vi "catch.vi"(11 "NXT/EV3":T1) -> (3 "NXT/EV3 2":T1)   [LabVIEW 2016]
uses:
  <vilib>/NXT/Subs/LVHSConnector.ctl
  <vilib>/NXT/LegoClasses/BrickReference/BrickReference.lvclass
  <vilib>/NXT/NXT Controls/ConnectionType.ctl
  <vilib>/NXT/Block Support/NXT_OutputPort.ctl
  <vilib>/NXT/NXTIO Xnodes/NXTIONodeSubVIs/NXTMoveMotors.vi
  <vilib>/NXT/Dual Mode Library/Waits/Wait_Num.vi
  <vilib>/NXT/NXTIO Xnodes/NXTIONodeSubVIs/NXTStopMotors.vi
  <vilib>/NXT/Dual Mode Library/Waits/Wait_Rotation.vi
  <vilib>/NXT/NXTIO Xnodes/AddressXNode/NXTIOAddress.xnode
  <vilib>/NXT/NXTIO Xnodes/NXTIOXNode/NXTIO.xnode
panel:
  in  "Numeric":dbl format="%#1.6f"
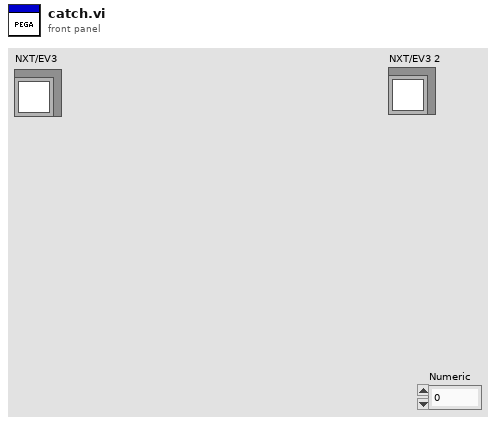
[diagram p1: front panel]
types:
  T1 = typedef "LVHSConnector.ctl" = refnum<class "BrickReference.lvclass">
  T2 = typedef "ConnectionType.ctl" = enum16{"Bluetooth", "USB", "WiFi"}
  T3 = typedef "NXT_OutputPort.ctl" = u8
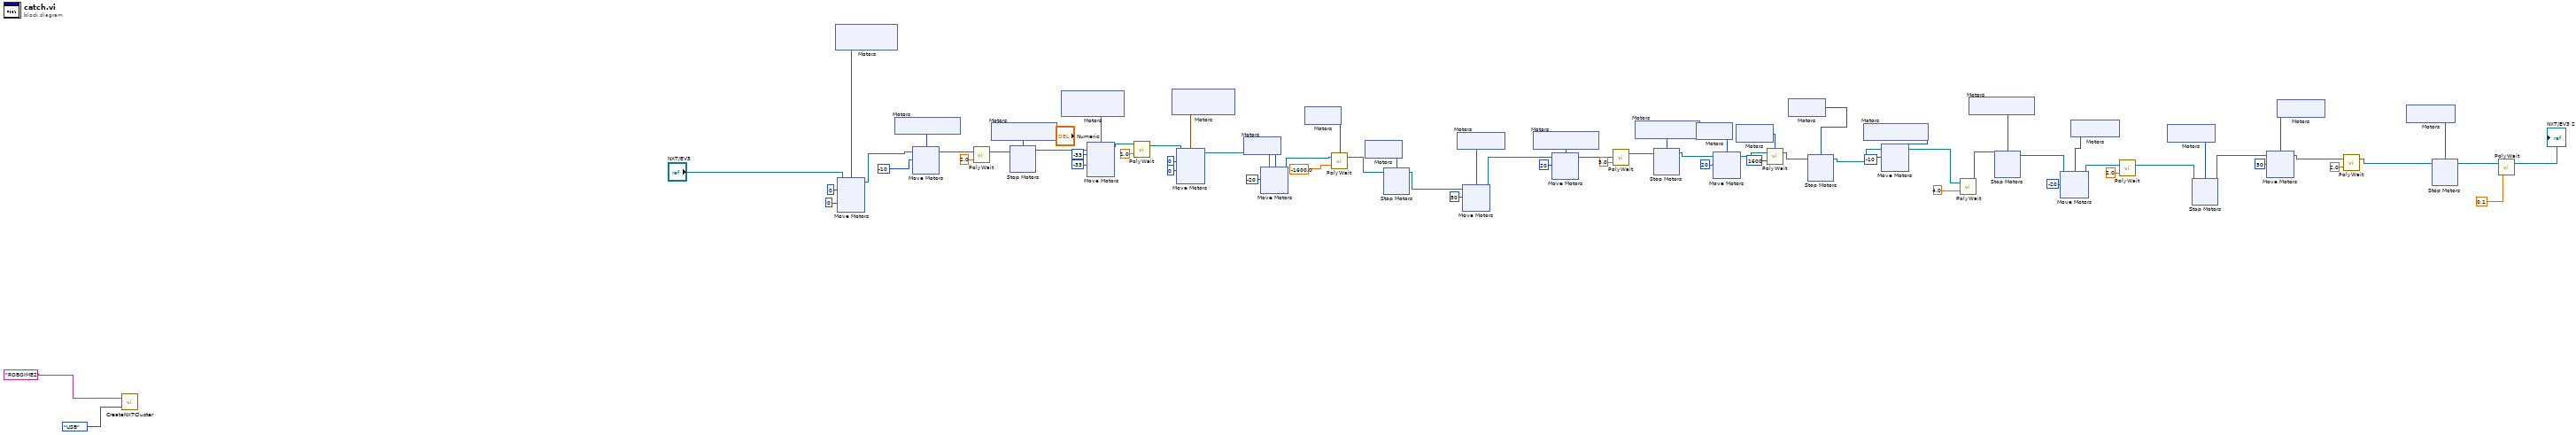
[diagram p0: block diagram]
diagram:
  n1 = call <vilib>:"CreateNXTCluster.vi"("Connection Type"=ConnectionType."USB", "NXT/EV3 name"="ROBOIME2") -> ()  [unwired: 2 in, 1 out]
  n2 = xnode "Motors"() -> ("Motor"=w20:cluster{"Port":T3, "Port":T3})
  n3 = xnode "Move Motors"("Power/Speed 2"=i8 0 ("Power/Speed 1"), "Power/Speed 1"=i8 0, "Motors"=w20, "NXT/EV3"="NXT/EV3") -> ("NXT/EV3"=w71:T1)
  n4 = xnode "Motors"() -> ("Motor"=w69:T3)
  n5 = xnode "Move Motors"("Power/Speed 1"=i8 -10, "Motors"=w69, "NXT/EV3"=w71) -> ("NXT/EV3"=w66:T1)
  n6 = call-poly <vilib>:"PolyWait.vi"("Time (1 sec)"=sgl 2.0, "NXT/EV3"=w66) -> ("NXT/EV3"=w65:T1)  [unwired: 2 in]
  n7 = xnode "Motors"() -> ("Motor"=w58:T3)
  n8 = xnode "Stop Motors"("Motors"=w58, "NXT/EV3"=w65) -> ("NXT/EV3"=w15:T1)
  n9 = xnode "Motors"() -> ("Motor"=w16:cluster{"Port":T3, "Port":T3})
  n10 = xnode "Move Motors"("Power/Speed 2"=i8 -33, "Power/Speed 1"=i8 -33, "Motors"=w16, "NXT/EV3"=w15) -> ("NXT/EV3"=w12:T1)
  n11 = call-poly <vilib>:"PolyWait.vi"("Time (1 sec)"=sgl 1.0, "NXT/EV3"=w12) -> ("NXT/EV3"=w10:T1)  [unwired: 2 in]
  n12 = xnode "Motors"() -> ("Motor"=w17:cluster{"Port":T3, "Port":T3})
  n13 = xnode "Move Motors"("Power/Speed 2"=i8 0, "Power/Speed 1"=i8 0, "Motors"=w17, "NXT/EV3"=w10) -> ("NXT/EV3"=w9:T1)
  n14 = xnode "Motors"() -> ("Motor"=w51:T3)
  n15 = xnode "Move Motors"("Power/Speed 1"=i8 -20, "Motors"=w51, "NXT/EV3"=w9) -> ("NXT/EV3"=w49:T1)
  n16 = xnode "Motors"() -> ("Motor"=w2:T3)
  n17 = call-poly <vilib>:"PolyWait.vi"("Position Change (180)"=sgl -1600.0 ("Time (1 sec)"), "NXT/EV3"=w49, "Port (Port A)"=w2) -> ("NXT/EV3"=w47:T1)  [unwired: 1 in]
  n18 = xnode "Motors"() -> ("Motor"=w48:T3)
  n19 = xnode "Stop Motors"("Motors"=w48, "NXT/EV3"=w47) -> ("NXT/EV3"=w31:T1)
  n20 = xnode "Motors"() -> ("Motor"=w39:T3)
  n21 = xnode "Move Motors"("Power/Speed 1"=i8 50, "Motors"=w39, "NXT/EV3"=w31) -> ("NXT/EV3"=w30:T1)
  n22 = xnode "Motors"() -> ("Motor"=w59:T3)
  n23 = xnode "Move Motors"("Power/Speed 1"=i8 20, "Motors"=w59, "NXT/EV3"=w30) -> ("NXT/EV3"=w63:T1)
  n24 = call-poly <vilib>:"PolyWait.vi"("Time (1 sec)"=sgl 5.0, "NXT/EV3"=w63) -> ("NXT/EV3"=w61:T1)  [unwired: 2 in]
  n25 = xnode "Motors"() -> ("Motor"=w60:T3)
  n26 = xnode "Stop Motors"("Motors"=w60, "NXT/EV3"=w61) -> ("NXT/EV3"=w45:T1)
  n27 = xnode "Motors"() -> ("Motor"=w46:T3)
  n28 = xnode "Move Motors"("Power/Speed 1"=i8 20, "Motors"=w46, "NXT/EV3"=w45) -> ("NXT/EV3"=w43:T1)
  n29 = xnode "Motors"() -> ("Motor"=w1:T3)
  n30 = call-poly <vilib>:"PolyWait.vi"("Position Change (180)"=1600, "NXT/EV3"=w43, "Port (Port A)"=w1) -> ("NXT/EV3"=w42:T1)  [unwired: 1 in]
  n31 = xnode "Motors"() -> ("Motor"=w29:T3)
  n32 = xnode "Stop Motors"("Motors"=w29, "NXT/EV3"=w42) -> ("NXT/EV3"=w41:T1)
  n33 = xnode "Motors"() -> ("Motor"=w40:T3)
  n34 = xnode "Move Motors"("Power/Speed 1"=i8 -10, "Motors"=w40, "NXT/EV3"=w41) -> ("NXT/EV3"=w55:T1)
  n35 = call-poly <vilib>:"PolyWait.vi"("Time (1 sec)"=sgl 4.0, "NXT/EV3"=w55) -> ("NXT/EV3"=w53:T1)  [unwired: 2 in]
  n36 = xnode "Motors"() -> ("Motor"=w52:T3)
  n37 = xnode "Stop Motors"("Motors"=w52, "NXT/EV3"=w53) -> ("NXT/EV3"=w26:T1)
  n38 = xnode "Motors"() -> ("Motor"=w27:T3)
  n39 = xnode "Move Motors"("Power/Speed 1"=i8 -20, "Motors"=w27, "NXT/EV3"=w26) -> ("NXT/EV3"=w24:T1)
  n40 = call-poly <vilib>:"PolyWait.vi"("Time (1 sec)"=sgl 2.0, "NXT/EV3"=w24) -> ("NXT/EV3"=w22:T1)  [unwired: 2 in]
  n41 = xnode "Motors"() -> ("Motor"=w23:T3)
  n42 = xnode "Stop Motors"("Motors"=w23, "NXT/EV3"=w22) -> ("NXT/EV3"=w21:T1)
  n43 = xnode "Motors"() -> ("Motor"=w37:T3)
  n44 = xnode "Move Motors"("Power/Speed 1"=i8 50, "Motors"=w37, "NXT/EV3"=w21) -> ("NXT/EV3"=w34:T1)
  n45 = call-poly <vilib>:"PolyWait.vi"("Time (1 sec)"=sgl 2.0, "NXT/EV3"=w34) -> ("NXT/EV3"=w32:T1)  [unwired: 2 in]
  n46 = xnode "Motors"() -> ("Motor"=w35:T3)
  n47 = xnode "Stop Motors"("Motors"=w35, "NXT/EV3"=w32) -> ("NXT/EV3"=w5:T1)
  n48 = call-poly <vilib>:"PolyWait.vi"("Time (1 sec)"=0.1, "NXT/EV3"=w5) -> ("NXT/EV3"=→"NXT/EV3 2":T1)  [unwired: 2 in]
